vi "Inverse Complex FFT PtByPt.vi"(2 "initialize":bool, 3 "sample length":i32=100, 5 "x":cdb format="%#.6g") -> (0 "error":i32, 1 "Inverse Complex FFT{X}":cdb[](array[numeric]))   [LabVIEW 2020, in "NI_PtbyPt.lvlib"]
doc: "Computes the inverse discrete Fourier transform (IDFT) of the set of input data points specified by <B>sample length</B>. This VI is similar to the Inverse FFT VI. Wire data to the <B>x</B> input to determine the polymorphic instance to use or manually select the instance."
uses:
  NI_PtbyPt.lvlib
  Ramp Pattern by Samples.vi
  NI_AALBase.lvlib
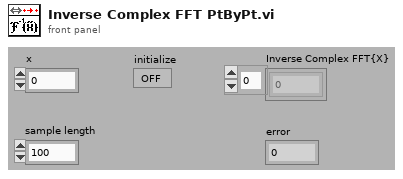
[diagram p1: front panel]
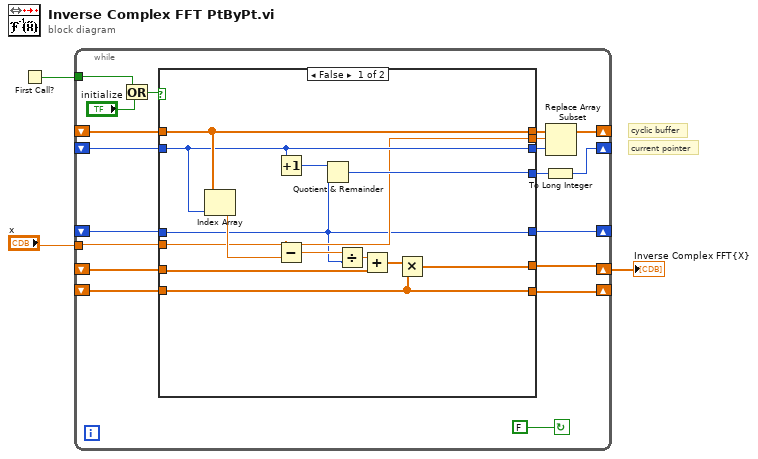
[diagram p0: block diagram]
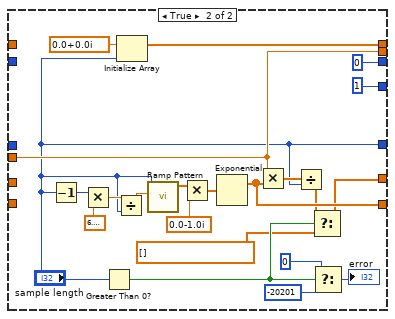
[diagram p2: hidden frame]
diagram:
  # "current pointer"
  # "cyclic buffer"
  n1 = First Call?() -> (First Call?: T/F=w1:bool)
  n2 = while {
    tunnel: w1 -> [w4]
    shift-left: _ -> [w10]
    shift-right: [w11] -> _
    shift-left: _ -> [w13]
    shift-right: [w12] -> _
    shift-left: _ -> [w18]
    shift-right: [w19] -> _
    tunnel: "x" -> [w9]
    shift-left: _ -> [w20]
    shift-right: [w22] -> w3
    shift-left: _ -> [w21]
    shift-right: [w16] -> _
    stop <- FALSE continue-if-true
    n3 = Or(x=w4, y="initialize") -> (x .or. y?=w5:bool)
    n4 = case shown="False" w5 {
      tunnel: w10 -> [w23 _]
      tunnel: [w29 w36] -> w22
      tunnel: [w35 w56] -> w17
      tunnel: w21 -> [w35 _]
      tunnel: w20 -> [w32 _]
      tunnel: [w30 w46] -> w19
      tunnel: w18 -> [w30 _]
      tunnel: [w33 0 ("Index")] -> w15
      tunnel: [w26 1 ("Index")] -> w14
      tunnel: w13 -> [w33 _]
      tunnel: [w23 "sample length"] -> w11
      tunnel: w9 -> [w25 w45]
      tunnel: [w25 w45] -> w8
      frame False {
        n5 = Index Array(array=w35, index=w33) -> (element=w34:cdb)
        n6 = Increment(x=w33) -> (x+1=w27:i32)
        n7 = Subtract(x=w25, y=w34) -> (x-y=w28:cdb)
        n8 = Quotient & Remainder(x=w27, y=w23) -> (x-y*floor(x/y)=w26:i32)  [unwired: 1 out]
        n9 = Divide(x=w28, y=w23) -> (x/y=w24:cdb)
        n10 = Add(x=w24, y=w32) -> (x+y=w31:cdb[])
        n11 = Multiply(x=w31, y=w30) -> (x*y=w29:cdb[])
      }
      frame True {
        n12 = Decrement(x="sample length") -> (x-1=w52:i32)
        n13 = Multiply(x=w52, y=6.283185307179586) -> (x*y=w51:dbl)
        n14 = Greater Than 0?(x="sample length") -> (x > 0?=w39:bool)
        n15 = Divide(x=w51, y="sample length") -> (x/y=w50:dbl)
        n16 = Initialize Array(cdb 0.0+0.0i ("Element Data"), "sample length") -> (w56:cdb[])
        n17 = call-poly "Ramp Pattern.vi"("end"=w50, "samples"="sample length") -> ("Ramp Pattern"=w53:dbl[])  [unwired: 8 in, 1 out]
        n18 = Multiply(x=w53, y=cdb 0.0-1.0i) -> (x*y=w47:cdb[])
        n19 = Exponential(1:w47) -> (0:w46:cdb[])
        n20 = Multiply(x=w45, y=w46) -> (x*y=w44:cdb[])
        n21 = Divide(x=w44, y="sample length") -> (x/y=w38:cdb[])
        n22 = Select(t=w38, s=w39, f=cdb[] []) -> (s? t:f=w36:cdb[])
        n23 = Select(t=0, s=w39, f=-20201) -> (s? t:f=→"error":i32)
      }
    }
    n24 = To Long Integer(number=w14) -> (32bit integer=w12:i32)
    n25 = Replace Array Subset(array=w17, new element=w8, index=w15) -> (w16:cdb[])
  }
  "Inverse Complex FFT{X}" <- w3
